vi "PresetPosition.vi"(8 "error in (no error)":errorcluster) -> (0 "error out (no error)":errorcluster)   [LabVIEW 2009]
uses:
  typedefs/AxisSelect_Enum.ctl
panel:
  out "Current Position":dbl caption="[mm]" format="%#.3g"
  in  "Cancel":bool
  in  "Apply":bool
  in  "OK":bool
  in  "Preset Position":dbl caption="[mm]"
  in  "Axis":T1
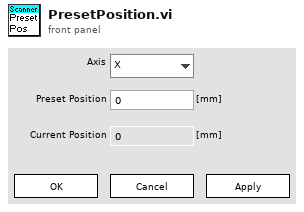
[diagram p1: front panel]
types:
  T1 = typedef "AxisSelect_Enum.ctl" = enum16{"X", "Y", "Z", "Axis Space"}
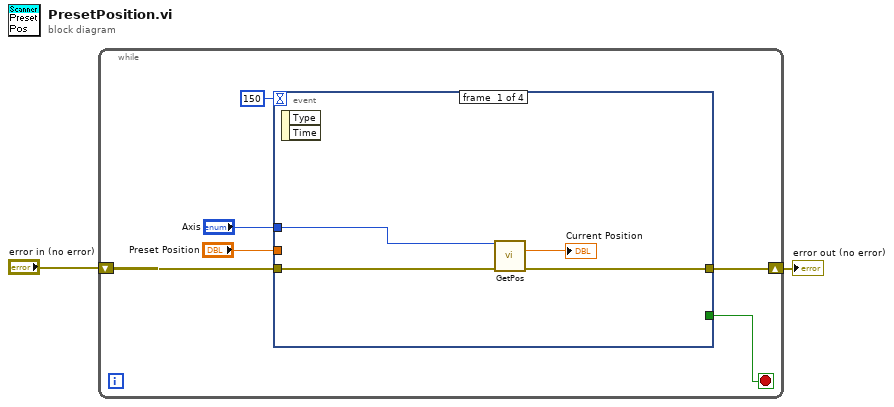
[diagram p0: block diagram]
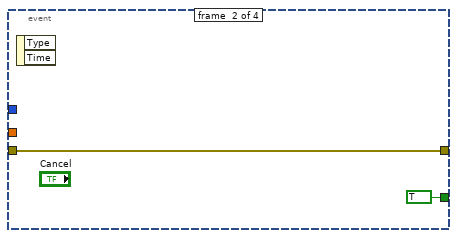
[diagram p2: hidden frame]
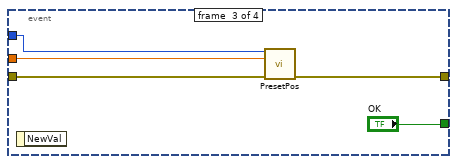
[diagram p3: hidden frame]
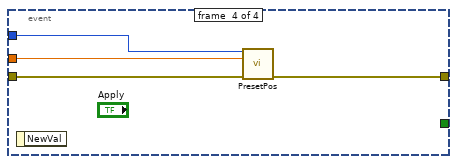
[diagram p4: hidden frame]
diagram:
  n1 = while {
    shift-right: [w4] -> w1
    shift-left: "error in (no error)" -> [w3]
    stop <- w8 stop-if-true
    n2 = event shown="[1] Panel Close;  \"Cancel\": Value Change" {
      selector: _ -> [_ _ _ _]
      dyn-events: _ -> [_ _ _ _]
      timeout: 150 -> [_ _ _ _]
      tunnel: [_ TRUE ("OK") "OK" _] -> w8
      tunnel: "Axis" -> [w11 _ w19 w23]
      tunnel: "Preset Position" -> [_ _ w18 w22]
      tunnel: [w10 w14 w15 w20] -> w4
      tunnel: w3 -> [w9 w14 w16 w21]
      event #0 {
        n3 = event-data() -> ()  [unwired: 1 in, 2 out]
        n4 = call "GetPos.vi"("Axis In"=w11, "error in (no error)"=w9) -> ("Position"=→"Current Position":dbl, "error out"=w10:errorcluster)  [unwired: 10 in, 2 out]
      }
      event #1 {
        n5 = event-data() -> ()  [unwired: 1 in, 2 out]
      }
      event #2 {
        n6 = event-data() -> ()  [unwired: 1 in, 1 out]
        n7 = call "PresetPos.vi"("Axis In (Axis Space)"=w19, "Preset Position"=w18, "error in (no error)"=w16) -> ("error out"=w15:errorcluster)  [unwired: 11 in, 1 out]
      }
      event #3 {
        n8 = event-data() -> ()  [unwired: 1 in, 1 out]
        n9 = call "PresetPos.vi"("Axis In (Axis Space)"=w23, "Preset Position"=w22, "error in (no error)"=w21) -> ("error out"=w20:errorcluster)  [unwired: 11 in, 1 out]
      }
    }
  }
  "error out (no error)" <- w1
